vi "Send Command.vi"(8 "error in":errorcluster, 9 "Value":variant, 10 "Command":string, 11 "SwitchMatrix in":refnum<class "SwitchMatrix.lvclass">) -> (0 "error out":errorcluster, 3 "SwitchMatrix out":refnum<class "SwitchMatrix.lvclass">)   [LabVIEW 2019, in "SwitchMatrix.lvlib" / "SwitchMatrix.lvclass"]
uses:
  Library/SwitchMatrix.lvclass
  C:/Users/Public/Documents/Development/builds/Engine/Engine.lvlibp/Project/Engine.lvclass
  SwitchMatrix Messages/Toggle Relay Msg/Toggle Relay Msg.lvclass/Toggle Relay Msg.ctl
  builds/Engine/Engine.lvlibp/Accessors/Read Self Q.vi
  builds/Engine/Actor Framework.lvlibp/1abvi3w/vi.lib/ActorFramework/Message Enqueuer/Enqueue.vi
  builds/Engine/Actor Framework.lvlibp/1abvi3w/vi.lib/ActorFramework/Message Enqueuer/Message Enqueuer.lvclass
  SwitchMatrix Messages/Toggle Relay Msg/Toggle Relay Msg.lvclass
  SwitchMatrix Messages/Open All Relays Msg/Open All Relays Msg.lvclass
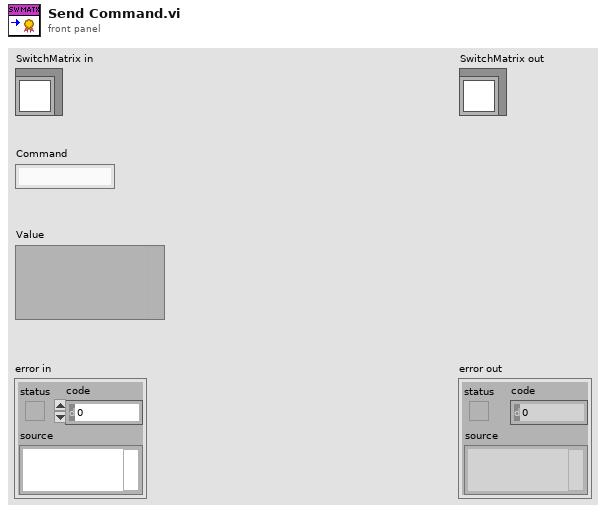
[diagram p1: front panel]
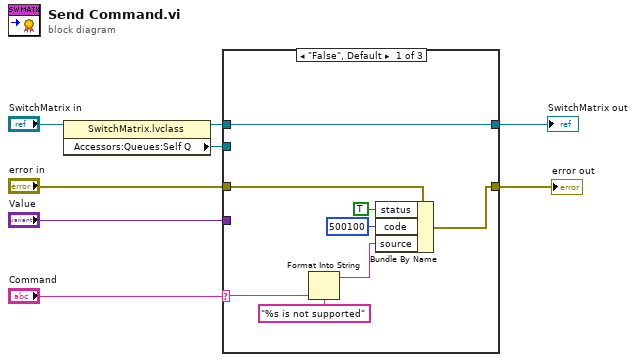
[diagram p0: block diagram]
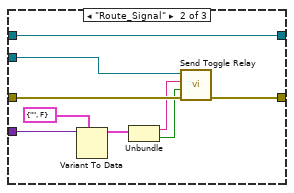
[diagram p2: hidden frame]
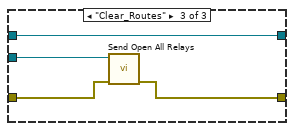
[diagram p3: hidden frame]
diagram:
  n1 = property class="SwitchMatrix.lvclass"(reference="SwitchMatrix in") -> (reference out=w5:refnum<class "SwitchMatrix.lvclass">, "Accessors:Queues:Self Q"=w6:refnum<class "Message Enqueuer.lvclass">)  [unwired: 1 in, 1 out]
  n2 = case shown="\"False\", Default" "Command" {
    selector: "Command" -> [w11 _ _]
    tunnel: w6 -> [_ w23 w29]
    tunnel: w5 -> [w16 w24 w26]
    tunnel: "Value" -> [_ w25 _]
    tunnel: [w16 w24 w26] -> w3
    tunnel: "error in" -> [w15 w22 w28]
    tunnel: [w14 w21 w27] -> w1
    frame "False", Default {
      n3 = Format Into String(format string="%s is not supported", w11) -> (resulting string=w9:string)  [unwired: 2 in, 1 out]
      n4 = Bundle By Name(cluster=w15, "status"=TRUE, "code"=500100, "source"=w9) -> (w14:errorcluster)
    }
    frame "Route_Signal" {
      n5 = Variant To Data(type=cluster{"Name":string, "State":bool} {"Name"="", "State"=FALSE}, Variant=w25) -> (data=w19:cluster{"Name":string, "State":bool})  [unwired: 1 in, 1 out]
      n6 = Unbundle(w19) -> ("Name"=w18:string, "State"=w17:bool)
      n7 = call "Send Toggle Relay.vi"("error in (no error)"=w22, "Relay State"=w17, "Relay Name"=w18, "Message Enqueuer"=w23) -> ("error out"=w21:errorcluster)  [unwired: 6 in, 1 out]
    }
    frame "Clear_Routes" {
      n8 = call "Send Open All Relays.vi"("error in (no error)"=w28, "Message Enqueuer"=w29) -> ("error out"=w27:errorcluster)  [unwired: 8 in, 1 out]
    }
  }
  "error out" <- w1
  "SwitchMatrix out" <- w3
